vi "EMPAS_7HP_Data.vi"() -> ()   [LabVIEW 2022 SP3]
uses:
  Data plotting/MATLAB/MATLAB_Mode.ctl
panel:
  in  "Probe offset Roll":dbl=3.8
  in  "Uref":dbl=34.4
  in  "Relative yaw (deg)":sgl
  out "Number of Measurements":i32
  in  "MATLAB Folder":path=path "C:/EnFlo Software MATLAB"
  out "array":string[][](array[string])
  in  "Data File":path=path "C:/EnFlo Software MATLAB/RUN086.csv"
  out "error out":errorcluster
  out "Error String":string
  in  "Calib Filename":string="20200214155940_7HP_1014.xls"
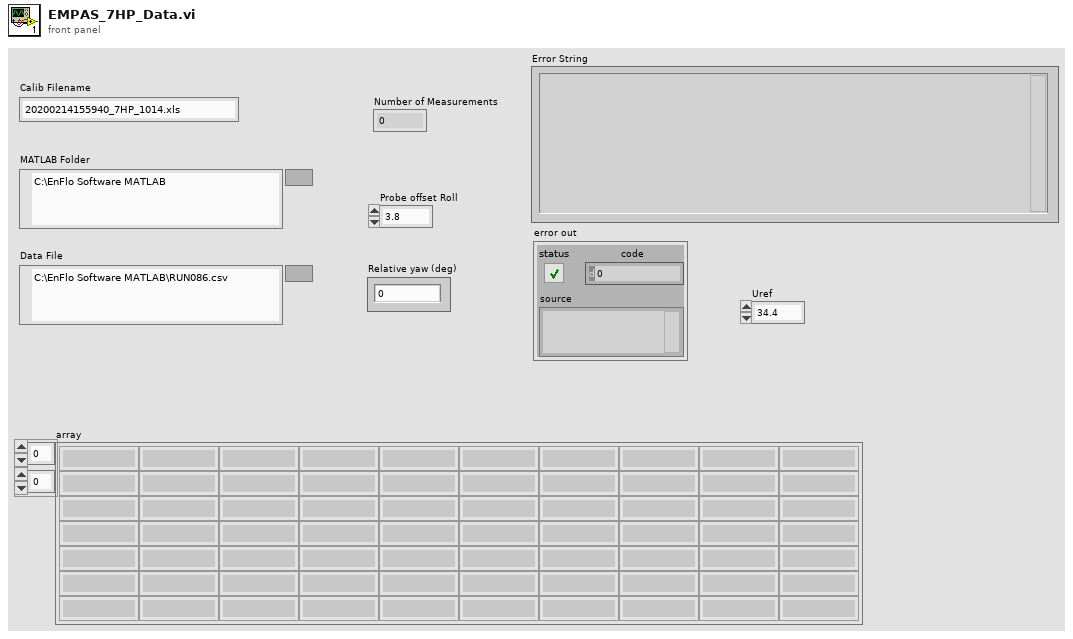
[diagram p1: front panel]
types:
  T1 = typedef "MATLAB_Mode.ctl" = enum16{"1D Plotter", "2D Plotter", "LP Plotter", "7HP UVW"}
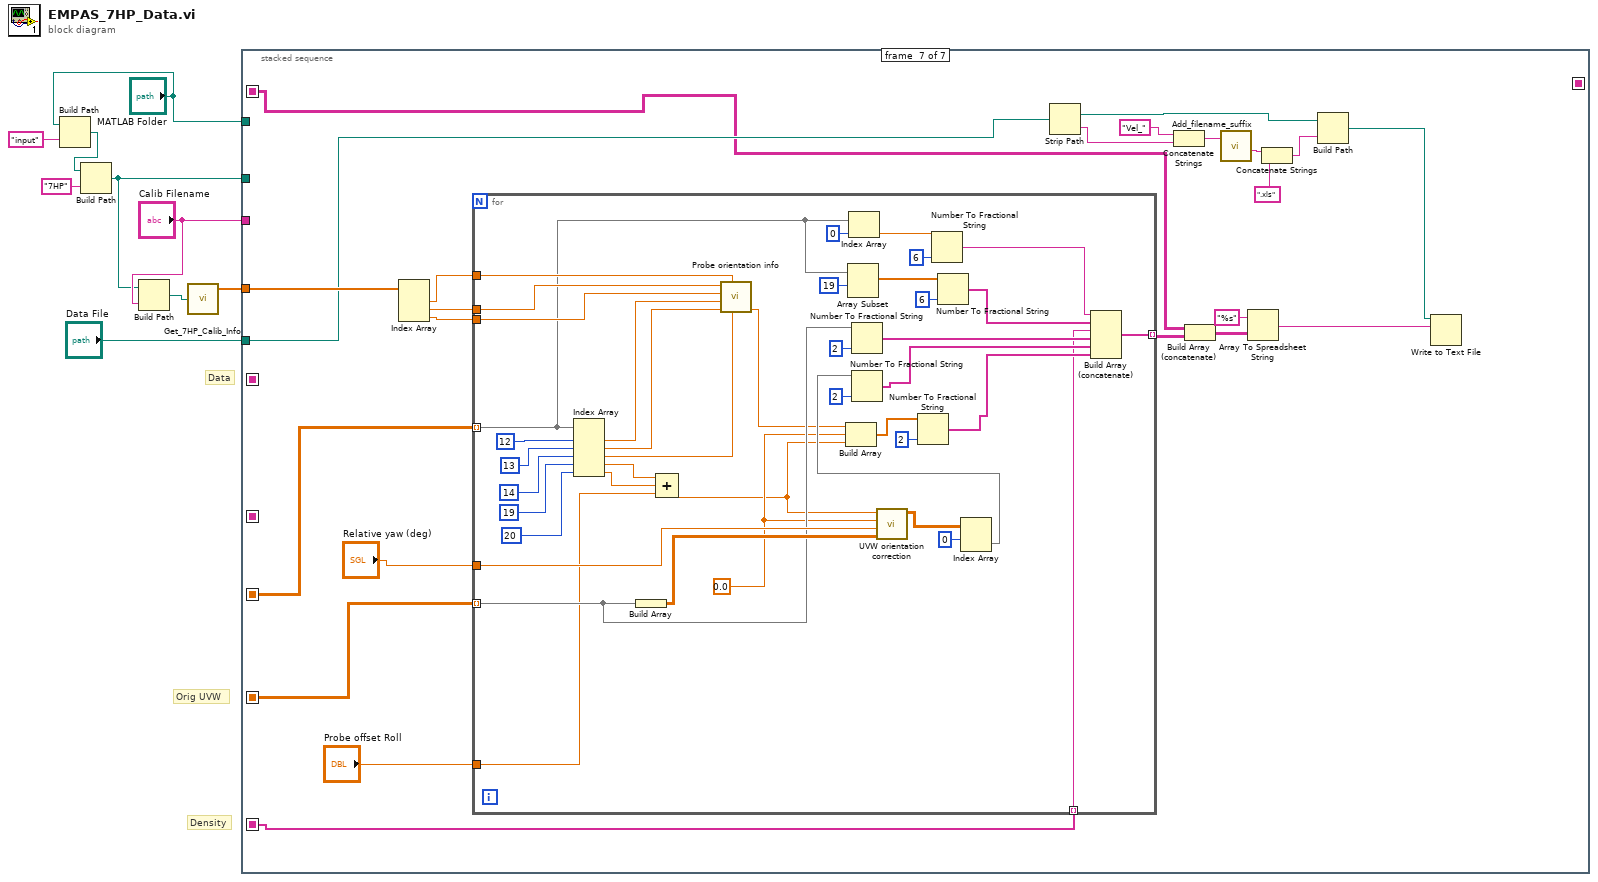
[diagram p0: block diagram]
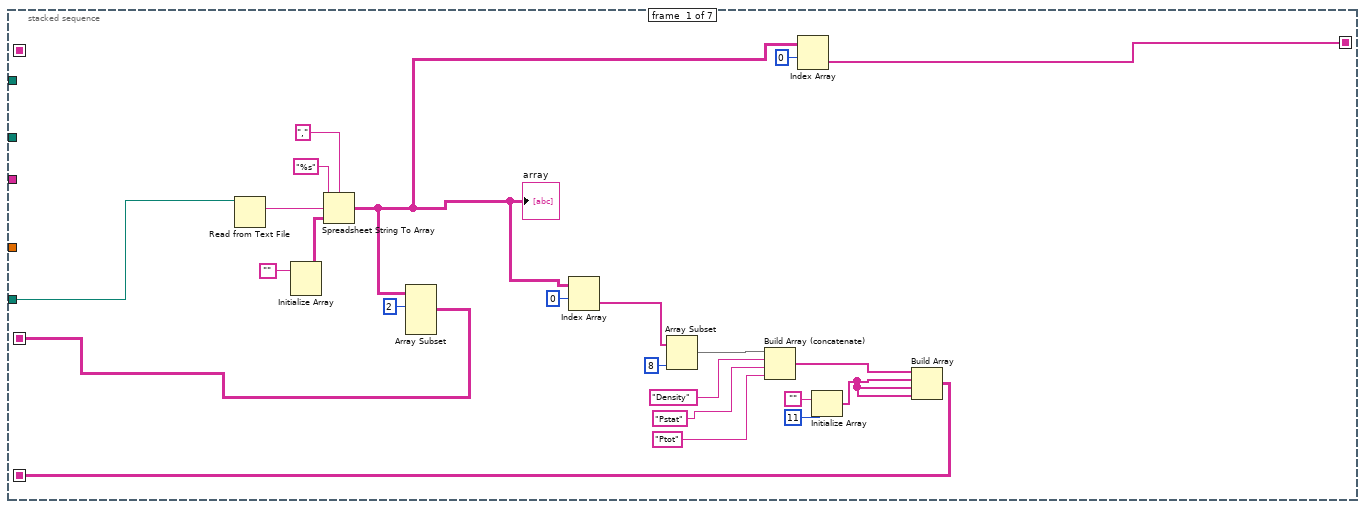
[diagram p2: hidden frame]
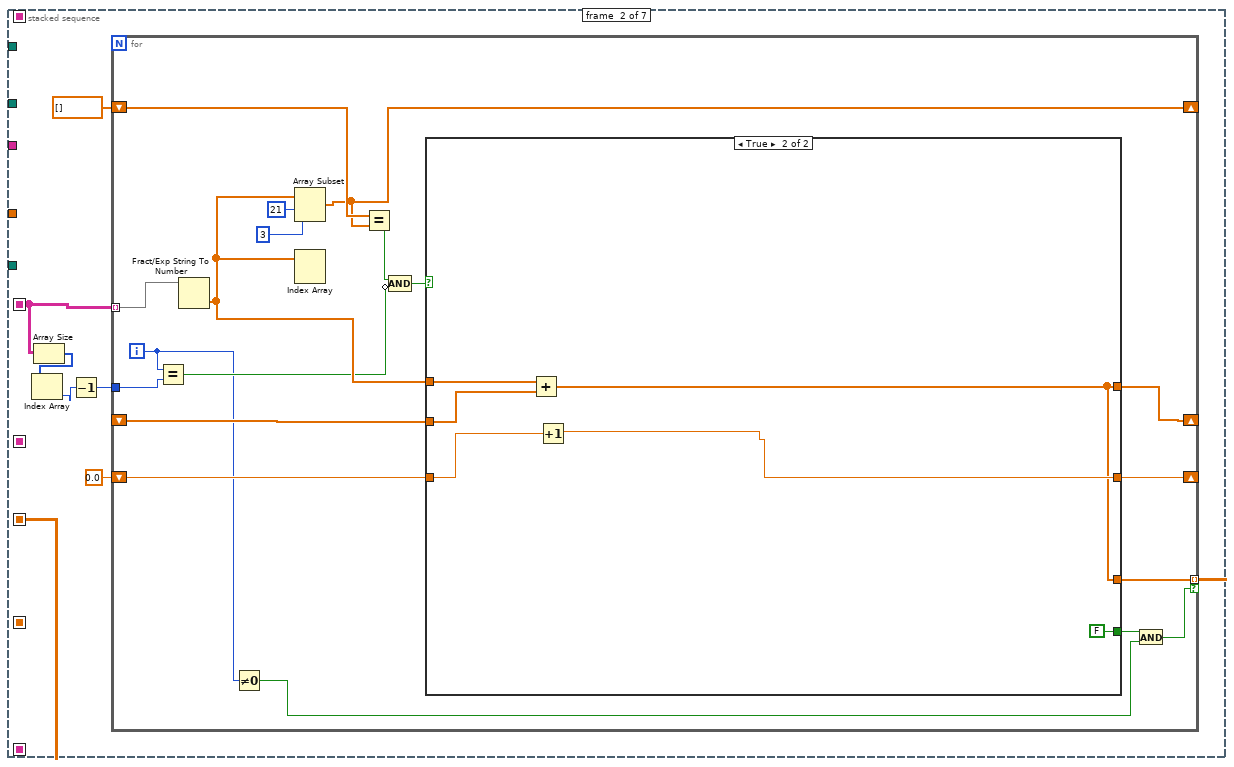
[diagram p3: hidden frame]
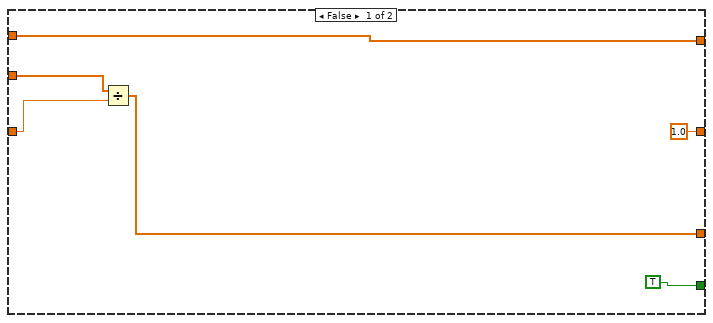
[diagram p4: hidden frame]
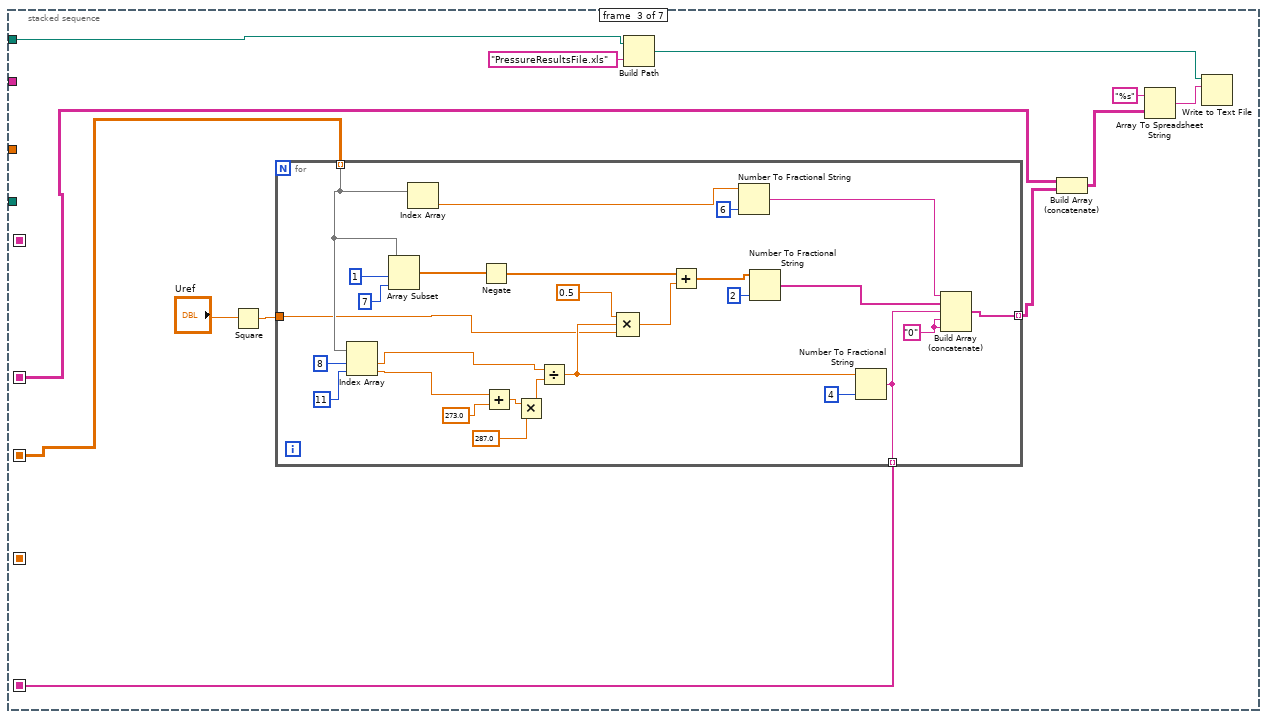
[diagram p5: hidden frame]
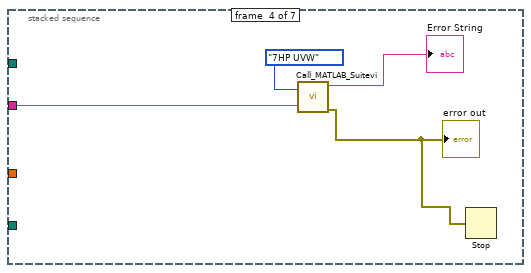
[diagram p6: hidden frame]
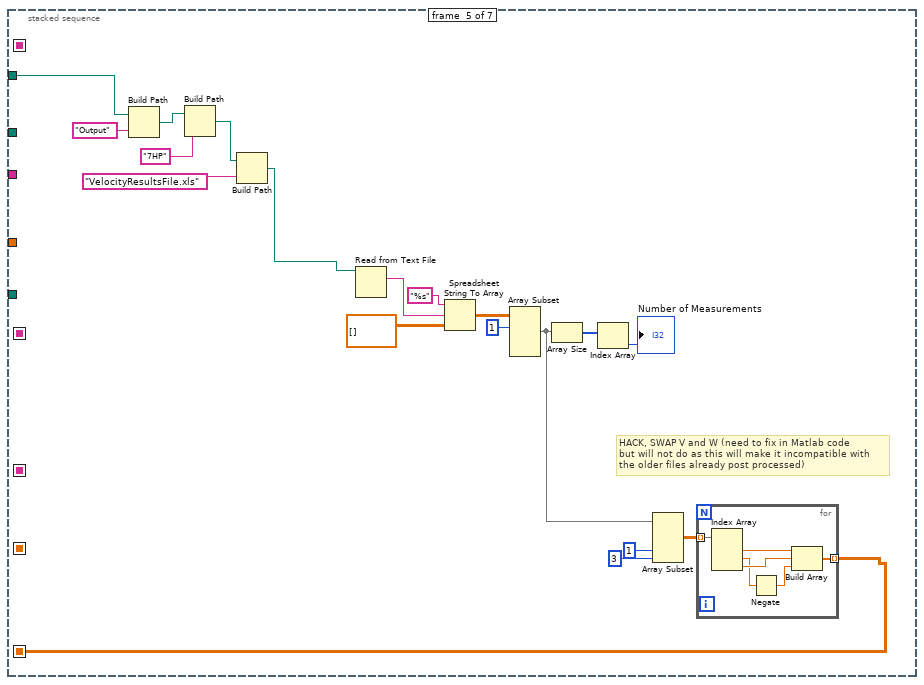
[diagram p7: hidden frame]
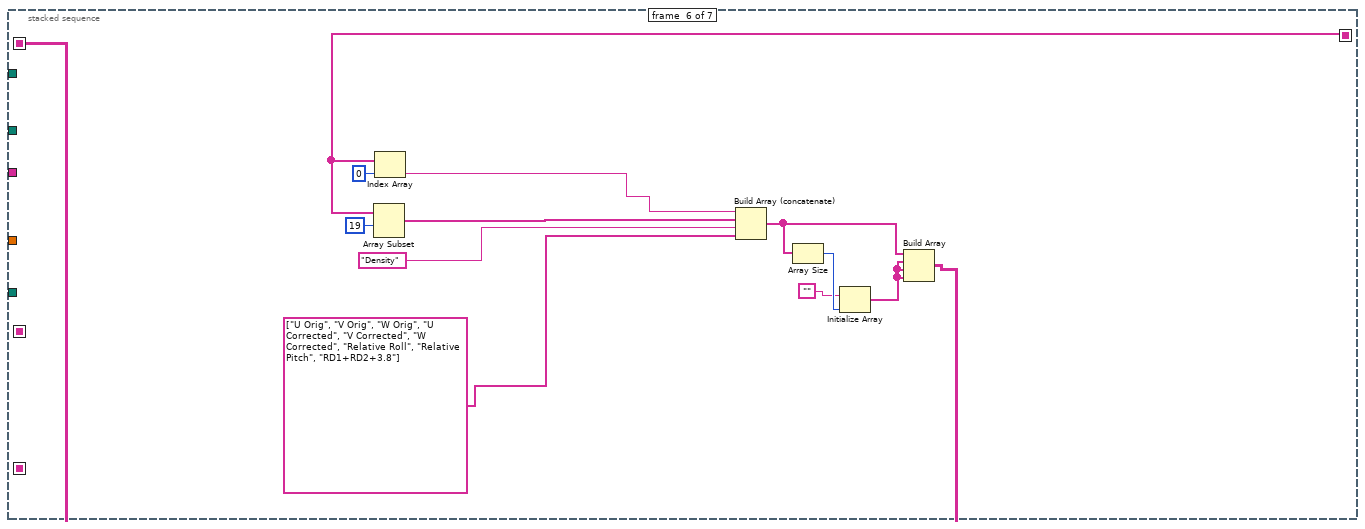
[diagram p8: hidden frame]
diagram:
  # "Density"
  # "Orig UVW"
  # "Data"
  n1 = Build Path(base path="MATLAB Folder", name or relative path="input") -> (appended path=w7:path)
  n2 = Build Path(base path=w7, name or relative path="7HP") -> (appended path=w4:path)
  n3 = Build Path(base path=w4, name or relative path="Calib Filename") -> (appended path=w3:path)
  n4 = call "Get_7HP_Calib_Info.vi"("Results file"=w3) -> ("ax ay az"=w2:sgl[])  [unwired: 2 out]
  n5 = stacked-sequence {
    seq-local: [w26 _ _ _ _ _ _] -> [_ w36 _ _ _ _ _]
    seq-local: [_ _ _ _ w114 _ _] -> [_ _ _ _ _ _ w168]
    seq-local: [_ _ w71 _ _ _ _] -> [_ _ _ _ _ _ w153]
    seq-local: [w11 _ _ _ _ _ _] -> [_ _ _ _ _ w148 _]
    seq-local: [_ _ _ _ _ w139 _] -> [_ _ _ _ _ _ w162]
    seq-local: [_ w37 _ _ _ _ _] -> [_ _ w81 _ _ _ w152]
    seq-local: [w10 _ _ _ _ _ _] -> [_ _ w74 _ _ _ _]
    tunnel: "MATLAB Folder" -> [_ _ _ _ w127 _ _]
    tunnel: "Calib Filename" -> [_ _ _ w110 _ _ _]
    tunnel: w4 -> [_ _ w78 _ _ _ _]
    tunnel: w2 -> [_ _ _ _ _ _ w173]
    tunnel: "Data File" -> [w14 _ _ _ _ _ w167]
    frame #0 {
      n6 = Read from Text File(file (use dialog)=w14) -> (text=w30:string)  [unwired: 3 in, 3 out]
      n7 = Initialize Array("") -> (w31:string[][])  [unwired: 2 in]
      n8 = Spreadsheet String To Array(delimiter (Tab)=",", format string="%s" ("delimiter (Tab)"), spreadsheet string=w30, array type (2D Dbl)=w31) -> (array=w13:string[][])
      "array" <- w13
      n9 = Array Subset(array=w13, index (row)=2 ("index")) -> (w26:string[][])  [unwired: 3 in]
      n10 = Index Array(array=w13, index (row)=0) -> (element=w23:string[])  [unwired: 1 in]
      n11 = Array Subset(array=w23, length=8) -> (w22:string[])  [unwired: 1 in]
      n12 = Build Array (concatenate)(w22, "Density", "Pstat", "Ptot") -> (w18:string[])
      n13 = Index Array(array=w13, index (row)=0) -> (element=w11:string[])  [unwired: 1 in]
      n14 = Initialize Array("", 11 ("dimension size")) -> (w15:string[])
      n15 = Build Array(w18, w15, w15, w15) -> (w10:string[][])
    }
    frame #1 {
      n16 = Array Size(array=w36) -> (size(s)=w35:i32[])
      n17 = Index Array(array=w35) -> (element=w34:i32)  [unwired: 1 in]
      n18 = Decrement(x=w34) -> (x-1=w33:i32)
      n19 = for {
        shift-right: [w51] -> _
        shift-left: _ -> [w52]
        tunnel: w36 -> [w58] mode=indexing
        shift-right: [w54] -> _
        shift-left: dbl[] [] -> [w55]
        shift-right: [w50] -> _
        shift-left: 0.0 -> [w49]
        tunnel: [w48] -> w37 mode=indexing if=w41
        tunnel: w33 -> [w47]
        i -> [w43]
        n20 = Equal?(x=w43, y=w47) -> (x = y?=w44:bool)
        n21 = Fract/Exp String To Number(string=w58) -> (number=w53:dbl[])  [unwired: 3 in, 1 out]
        n22 = Not Equal To 0?(x=w43) -> (x != 0?=w40:bool)
        n23 = Array Subset(array=w53, index=21, length=3) -> (w54:dbl[])
        n24 = Index Array(array=w53) -> ()  [unwired: 2 in, 2 out]
        n25 = Equal?(x=w55, y=w54) -> (x = y?=w46:bool)
        n26 = Compound Arithmetic op=AND(w46, invert w44) -> (w45:bool)
        n27 = case shown="True" w45 {
          tunnel: w53 -> [w62 w70]
          tunnel: w52 -> [w64 w69]
          tunnel: [w62 w65] -> w51
          tunnel: [1.0 w68] -> w50
          tunnel: w49 -> [w63 w67]
          tunnel: [w61 w65] -> w48
          tunnel: [TRUE FALSE] -> w42
          frame False {
            n28 = Divide(x=w64, y=w63) -> (x/y=w61:dbl[])
          }
          frame True {
            n29 = Add(x=w70, y=w69) -> (x+y=w65:dbl[])
            n30 = Increment(x=w67) -> (x+1=w68:dbl)
          }
        }
        n31 = And(x=w42, y=w40) -> (x .and. y?=w41:bool)
      }
    }
    frame #2 {
      n32 = Square(x="Uref") -> (x^2=w82:dbl)
      n33 = for {
        tunnel: w81 -> [w98] mode=indexing
        tunnel: [w100] -> w75 mode=indexing
        tunnel: [w99] -> w71 mode=indexing
        tunnel: w82 -> [w94]
        w101 = "0"
        n34 = Index Array(array=w98, index #1=8 ("disabled index (col)"), index #2=11 ("index")) -> (element #1=w87:dbl, element #2=w86:dbl)
        n35 = Array Subset(array=w98, index=1, length=7) -> (w88:dbl[])
        n36 = Index Array(array=w98) -> (element=w84:dbl)  [unwired: 1 in]
        n37 = Negate(x=w88) -> (-x=w92:dbl[])
        n38 = Add(x=w86, y=273.0) -> (x+y=w106:dbl)
        n39 = Multiply(x=w106, y=287.0) -> (x*y=w104:dbl)
        n40 = Divide(x=w87, y=w104) -> (x/y=w96:dbl)
        n41 = Compound Arithmetic op=MULTIPLY(0.5, w96, w94) -> (w93:dbl)
        n42 = Add(x=w92, y=w93) -> (x+y=w91:dbl[])
        n43 = Number To Fractional String(number=w84, precision (6)=i16 6) -> (F-format string=w83:string)  [unwired: 2 in]
        n44 = Number To Fractional String(number=w91, precision (6)=i16 2) -> (F-format string=w89:string[])  [unwired: 2 in]
        n45 = Number To Fractional String(number=w96, precision (6)=i16 4) -> (F-format string=w99:string)  [unwired: 2 in]
        n46 = Build Array (concatenate)(w83, w89, w99, w101, w101) -> (w100:string[])
      }
      n47 = Build Path(base path=w78, name or relative path="PressureResultsFile.xls") -> (appended path=w72:path)
      n48 = Build Array (concatenate)(w74, w75) -> (w73:string[][])
      n49 = Array To Spreadsheet String(array=w73, 3:"%s" ("format string")) -> (spreadsheet string=w77:string)  [unwired: 1 in]
      n50 = Write to Text File(file (use dialog)=w72, text=w77) -> ()  [unwired: 2 in, 3 out]
    }
    frame #3 {
      n51 = call "Call_MATLAB_Suitevi.vi"("Mode"=MATLAB_Mode."7HP UVW", "Input String"=w110) -> ("Error String"=→"Error String":string, "error out"=w111:errorcluster)  [unwired: 2 out]
      "error out" <- w111
      n52 = Stop(stop? (T)=w111) -> ()
    }
    frame #4 {
      # "HACK, SWAP V and W (need to fix in Matlab code\nbut will not do as this will make it incompatible with\nthe older files already post processed)"
      n53 = Build Path(base path=w127, name or relative path="Output") -> (appended path=w129:path)
      n54 = Build Path(base path=w129, name or relative path="7HP") -> (appended path=w132:path)
      n55 = Build Path(base path=w132, name or relative path="VelocityResultsFile.xls") -> (appended path=w121:path)
      n56 = Read from Text File(file (use dialog)=w121) -> (text=w122:string)  [unwired: 3 in, 3 out]
      n57 = Spreadsheet String To Array(format string="%s", spreadsheet string=w122, array type (2D Dbl)=sgl[][] []) -> (array=w116:sgl[][])  [unwired: 1 in]
      n58 = Array Subset(array=w116, index (row)=1 ("index")) -> (w115:sgl[][])  [unwired: 3 in]
      n59 = Array Size(array=w115) -> (size(s)=w123:i32[])
      n60 = Index Array(array=w123) -> (element=→"Number of Measurements":i32)  [unwired: 1 in]
      n61 = Array Subset(array=w115, index (col)=1 ("index"), length (col)=3 ("length")) -> (w119:sgl[][])  [unwired: 2 in]
      n62 = for {
        tunnel: w119 -> [w138] mode=indexing
        tunnel: [w136] -> w114 mode=indexing
        n63 = Index Array(array=w138) -> (element #1=w137:sgl, element #2=w134:sgl, element #3=w135:sgl)  [unwired: 3 in]
        n64 = Negate(x=w134) -> (-x=w133:sgl)
        n65 = Build Array(w137, w135, w133) -> (w136:sgl[])
      }
    }
    frame #5 {
      n66 = Array Subset(array=w148, index=19) -> (w147:string[])  [unwired: 1 in]
      n67 = Index Array(array=w148, index=0) -> (element=w144:string)
      n68 = Build Array (concatenate)(w144, w147, "Density" ("element"), string[] ["U Orig", "V Orig", "W Orig", "U Corrected", "V Corrected", "W Corrected", "Relative Roll", "Relative Pitch", "RD1+RD2+3.8"] ("subarray")) -> (w141:string[])
      n69 = Array Size(array=w141) -> (size(s)=w143:i32)
      n70 = Initialize Array("", w143) -> (w140:string[])
      n71 = Build Array(w141, w140, w140, w140) -> (w139:string[][])
    }
    frame #6 {
      n72 = Index Array(array=w173) -> (element #1=w172:sgl, element #2=w171:sgl, element #3=w170:sgl)  [unwired: 3 in]
      n73 = for {
        tunnel: w172 -> [w214]
        tunnel: w171 -> [w213]
        tunnel: w170 -> [w212]
        tunnel: w152 -> [w202] mode=indexing
        tunnel: "Relative yaw (deg)" -> [w208]
        tunnel: w168 -> [w201] mode=indexing
        tunnel: [w191] -> w163 mode=indexing
        tunnel: w153 -> [w190] mode=indexing
        tunnel: "Probe offset Roll" -> [w175]
        w180 = sgl 0.0 ("Relative pitch (deg)")
        n74 = Index Array(array=w202, index #1=12 ("index"), index #2=13 ("index"), index #3=14 ("index"), index #4=19 ("index"), index #5=20 ("index")) -> (element #1=w189:dbl, element #2=w188:dbl, element #3=w187:dbl, element #4=w177:dbl, element #5=w176:dbl)
        n75 = Build Array(w201) -> (w207:sgl[][])
        n76 = Compound Arithmetic op=ADD(w177, w176, w175) -> (w174:dbl)
        n77 = call "Probe orientation info.vi"("az"=w187, "ax_cal"=w214, "ay"=w188, "ax"=w189, "az_cal"=w212, "ay_cal"=w213) -> ("Relative roll (deg)"=w194:sgl)  [unwired: 5 out]
        n78 = Build Array(w194, w180, w174) -> (w193:dbl[])
        n79 = Array Subset(array=w202, index=19) -> (w182:dbl[])  [unwired: 1 in]
        n80 = Index Array(array=w202, index=0) -> (element=w185:dbl)
        n81 = Number To Fractional String(number=w201, precision (6)=i16 2) -> (F-format string=w199:string[])  [unwired: 2 in]
        n82 = call "UVW orientation correction.vi"("(U, V, W) array in"=w207, "Relative yaw (deg)"=w208, "Relative pitch (deg)"=w180, "Relative roll (deg)"=w174) -> ("(U, V, W) array out"=w206:sgl[][])  [unwired: 5 in]
        n83 = Number To Fractional String(number=w193, precision (6)=i16 2) -> (F-format string=w192:string[])  [unwired: 2 in]
        n84 = Number To Fractional String(number=w185, precision (6)=i16 6) -> (F-format string=w184:string)  [unwired: 2 in]
        n85 = Number To Fractional String(number=w182, precision (6)=i16 6) -> (F-format string=w181:string[])  [unwired: 2 in]
        n86 = Index Array(array=w206, index (row)=0) -> (element=w197:sgl[])  [unwired: 1 in]
        n87 = Number To Fractional String(number=w197, precision (6)=i16 2) -> (F-format string=w196:string[])  [unwired: 2 in]
        n88 = Build Array (concatenate)(w184, w181, w190, w199, w196, w192) -> (w191:string[])
      }
      n89 = Strip Path(path=w167) -> (stripped path=w164:path, name=w166:string)
      n90 = Concatenate Strings("Vel_" ("string"), w166) -> (w157:string)
      n91 = Build Array (concatenate)(w162, w163) -> (w161:string[][])
      n92 = call "Add_filename_suffix.vi"("Filename"=w157) -> ("Base name"=w156:string)  [unwired: 1 in, 3 out]
      n93 = Array To Spreadsheet String(array=w161, 3:"%s" ("format string")) -> (spreadsheet string=w158:string)  [unwired: 1 in]
      n94 = Concatenate Strings(w156, ".xls" ("Suffix to add")) -> (w154:string)
      n95 = Build Path(base path=w164, name or relative path=w154) -> (appended path=w159:path)
      n96 = Write to Text File(file (use dialog)=w159, text=w158) -> ()  [unwired: 2 in, 3 out]
    }
  }
